vi "ATF-File & Folder.vi"(8 "error in (no error)":errorcluster) -> (0 "error out":errorcluster, 3 "File Output":T1)   [LabVIEW 2022 SP3]
uses:
  Controls/SeCrTs-file folder ctl.ctl
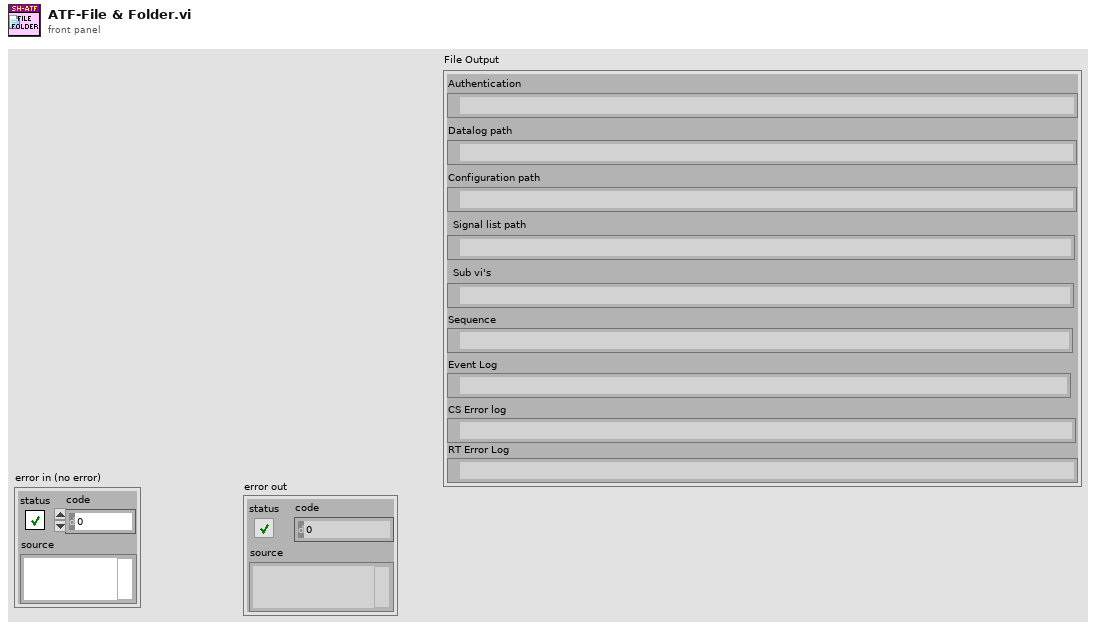
[diagram p1: front panel]
types:
  T1 = typedef "SeCrTs-file folder ctl.ctl" = cluster{"Datalog path":path, "Configuration path":path, "Signal list path":path, "Sub vi's":path, "Authentication":path, "Sequence":path, "Event Log":path, "CS Error log":path, "RT Error Log":path}
  T2 = enum32{"invalid app kind", "Development System", "Run Time System", "Student Edition", "Embedded LabVIEW", "Evaluation", "Custom"}
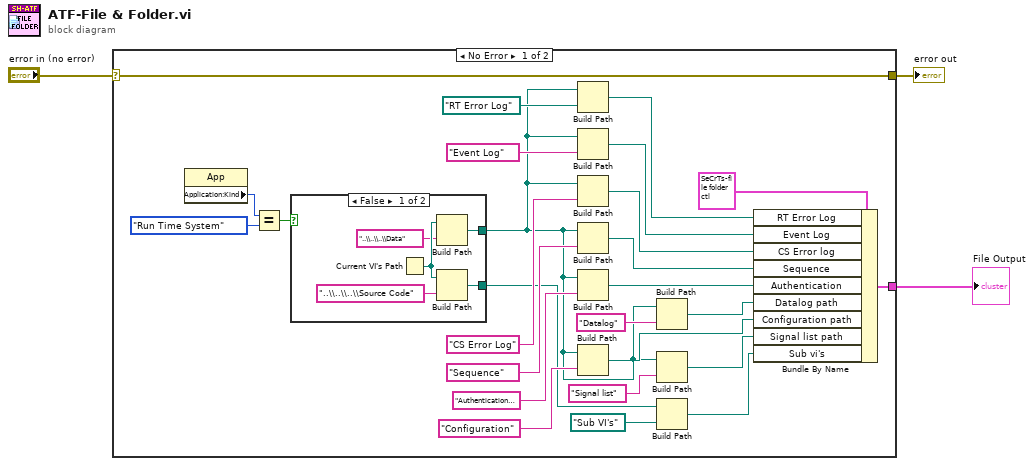
[diagram p0: block diagram]
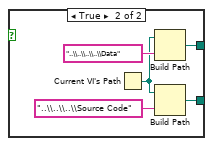
[diagram p2: hidden frame]
diagram:
  n1 = case shown="No Error" "error in (no error)" {
    selector: "error in (no error)" -> [w23 _]
    tunnel: [w23 _] -> w2
    tunnel: [w22 _] -> w1
    frame No Error {
      n2 = property class="App"() -> ("Application:Kind"=w29:T2)  [unwired: 2 in, 2 out]
      n3 = Equal?(x=w29, y=T2."Run Time System") -> (x = y?=w27:bool)
      n4 = case shown="False" w27 {
        tunnel: [w31 w35] -> w5
        tunnel: [w30 w38] -> w4
        frame False {
          n5 = Current VI's Path() -> (path=w34:path)
          n6 = Build Path(base path=w34, name or relative path="..\\..\\..\\Data") -> (appended path=w30:path)
          n7 = Build Path(base path=w34, name or relative path="..\\..\\..\\Source Code") -> (appended path=w31:path)
        }
        frame True {
          n8 = Current VI's Path() -> (path=w37:path)
          n9 = Build Path(base path=w37, name or relative path="..\\..\\..\\..\\Data") -> (appended path=w38:path)
          n10 = Build Path(base path=w37, name or relative path="..\\..\\..\\Source Code") -> (appended path=w35:path)
        }
      }
      n11 = Build Path(base path=w4, name or relative path=path "RT Error Log") -> (appended path=w6:path)
      n12 = Build Path(base path=w4, name or relative path="Event Log") -> (appended path=w9:path)
      n13 = Build Path(base path=w4, name or relative path="CS Error Log") -> (appended path=w8:path)
      n14 = Build Path(base path=w4, name or relative path="Sequence") -> (appended path=w12:path)
      n15 = Build Path(base path=w4, name or relative path="Authentication Details") -> (appended path=w14:path)
      n16 = Build Path(base path=w4, name or relative path="Configuration") -> (appended path=w19:path)
      n17 = Build Path(base path=w4, name or relative path="Datalog") -> (appended path=w24:path)
      n18 = Build Path(base path=w4, name or relative path="Signal list") -> (appended path=w18:path)
      n19 = Build Path(base path=w5, name or relative path=path "Sub VI's") -> (appended path=w16:path)
      n20 = Bundle By Name(cluster=T1 {"Datalog path"=path "", "Configuration path"=path "", "Signal list path"=path "", "Sub vi's"=path "", "Authentication"=path "", "Sequence"=path "", "Event Log"=path "", "CS Error log"=path "", "RT Error Log"=path ""} ("Cluster"), "RT Error Log"=w6, "Event Log"=w9, "CS Error log"=w8, "Sequence"=w12, "Authentication"=w14, "Datalog path"=w24, "Configuration path"=w19, "Signal list path"=w18, "Sub vi's"=w16) -> (w22:T1)
    }
    frame Error {
    }
  }
  "error out" <- w2
  "File Output" <- w1
